vi "Is Zombie.vi"(8 "Error In":errorcluster, 11 "GObject In":refnum<vi>) -> (0 "Error Out":errorcluster, 2 "Zombie?":bool, 3 "GObject Out":refnum<vi>)   [LabVIEW 2017, in "Toolkit.lvlib"]
doc: "Checks if a grave has a zombie (enabled corpse frame). A zombie is a Diagram Disable Structure with its legacy code frame (corpse) enabled."
uses:
  Toolkit.lvlib
  Typedefs/Grave Frames.ctl
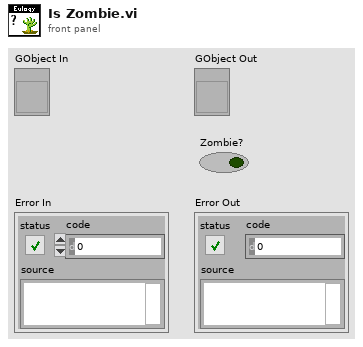
[diagram p1: front panel]
types:
  T1 = typedef "Toolkit.lvlib/Grave Frames.ctl" = enum16{"Corpse", "Spirit"}
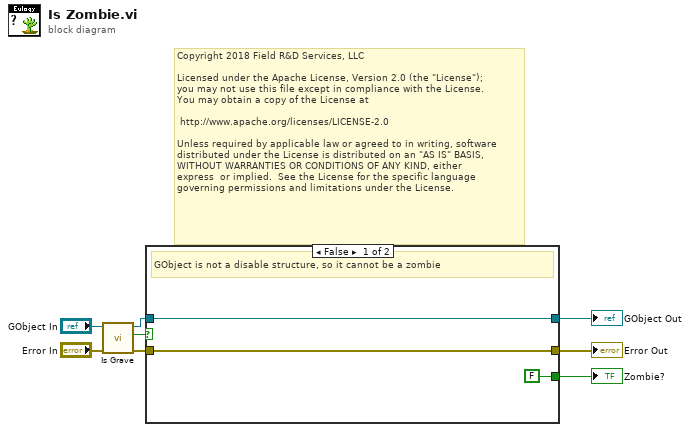
[diagram p0: block diagram]
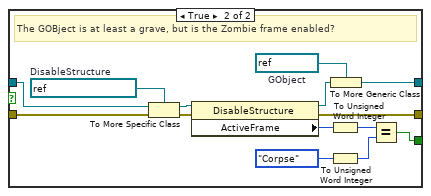
[diagram p2: hidden frame]
diagram:
  # "Copyright 2018 Field R&D Services, LLC\n\nLicensed under the Apache License, Version 2.0 (the \"License\");\nyou may not use this file except in compliance with the License.\nYou may obtain a copy of the License at\n\n\thttp://www.apache.org/licenses/LICENSE-2.0\n\nUnless required by applicable law or agreed to in writing, software\ndistributed under the License is distributed on an \"AS IS\" BASIS,\nWITHOUT WARRANTIES OR CONDITIONS OF ANY KIND, either \nexpress  or implied.  See the License for the specific language \ngoverning permissions and limitations under the License."
  n1 = call "Is Grave.vi"("Error In"="Error In", "GObject In"="GObject In") -> ("Error Out"=w4:errorcluster, "Grave?"=w5:bool, "GObject Out"=w3:refnum<vi>)  [unwired: 7 in]
  n2 = case shown="False" w5 {
    tunnel: [FALSE w16] -> w8
    tunnel: w4 -> [w10 w22]
    tunnel: w3 -> [w9 w25]
    tunnel: [w10 w15] -> w2
    tunnel: [w9 w21] -> w1
    frame False {
      # "GObject is not a disable structure, so it cannot be a zombie"
    }
    frame True {
      w20 = refnum<vi> refnum  # GObject
      w23 = refnum<vi> refnum  # DisableStructure
      # "The GOBject is at least a grave, but is the Zombie frame enabled?"
      n3 = To More Specific Class(target class=w23, reference=w25, error in=w22) -> (specific class reference=w24:refnum<vi>, error out=w18:errorcluster)
      n4 = property class="DisableStructure"(reference=w24, error in=w18) -> (reference out=w19:refnum<vi>, error out=w15:errorcluster, "ActiveFrame"=w17:i16)
      n5 = To Unsigned Word Integer(number=w17) -> (unsigned 16bit integer=w14:u16)
      n6 = To Unsigned Word Integer(number=Grave_Frames."Corpse" ("Frame")) -> (unsigned 16bit integer=w12:u16)
      n7 = To More Generic Class(target class=w20, reference=w19) -> (generic class reference=w21:refnum<vi>)
      n8 = Equal?(x=w14, y=w12) -> (x = y?=w16:bool)
    }
  }
  "Zombie?" <- w8
  "GObject Out" <- w1
  "Error Out" <- w2
